vi "BuildM3Sequence.vi"(8 "error in (no error)":errorcluster, 9 "Mode3 Test Properties":T2, 10 "Horizontal T deg":dbl=0.076 format="%#_13g", 11 "Sequence in":refnum<class "Sequence.lvclass">) -> (0 "error out":errorcluster, 2 "PAARD Test Sequence":T4[](array[typedef])=[{"StepType"=enum."Motion", "RF In/Out"=enum."Rx - RF Out", "Module/Raster"=0, "Polarization"=enum."Horizontal", "AO-64 Array"=[], "Position"=[]}, {"StepType"=enum."RasterTest", "RF In/Out"=enum."Tx - RF In", "Module/Raster"=0, "Polarization"=enum."Vertical", "AO-64 Array"=[], "Position"=[]}, {"StepType"=enum."Motion", "RF In/Out"=enum."Rx - RF Out", "Module/Raster"=1, "Polarization"=enum."Horizontal", "AO-64 Array"=[], "Position"=[]}, {"StepType"=enum."RasterTest", "RF In/Out"=enum."Tx - RF In", "Module/Raster"=0, "Polarization"=enum."Vertical", "AO-64 Array"=[], "Position"=[]}, {"StepType"=enum."Motion", "RF In/Out"=enum."Rx - RF Out", "Module/Raster"=2, "Polarization"=enum."Horizontal", "AO-64 Array"=[], "Position"=[]}, {"StepType"=enum."RasterTest", "RF In/Out"=enum."Tx - RF In", "Module/Raster"=0, "Polarization"=enum."Vertical", "AO-64 Array"=[], "Position"=[]}, {"StepType"=enum."Motion", "RF In/Out"=enum."Rx - RF Out", "Module/Raster"=3, "Polarization"=enum."Horizontal", "AO-64 Array"=[], "Position"=[]}, {"StepType"=enum."RasterTest", "RF In/Out"=enum."Tx - RF In", "Module/Raster"=0, "Polarization"=enum."Vertical", "AO-64 Array"=[], "Position"=[]}, {"StepType"=enum."Motion", "RF In/Out"=enum."Rx - RF Out", "Module/Raster"=4, "Polarization"=enum."Horizontal", "AO-64 Array"=[], "Position"=[]}, {"StepType"=enum."RasterTest", "RF In/Out"=enum."Tx - RF In", "Module/Raster"=0, "Polarization"=enum."Vertical", "AO-64 Array"=[], "Position"=[]}, {"StepType"=enum."Motion", "RF In/Out"=enum."Rx - RF Out", "Module/Raster"=5, "Polarization"=enum."Horizontal", "AO-64 Array"=[], "Position"=[]}, {"StepType"=enum."RasterTest", "RF In/Out"=enum."Tx - RF In", "Module/Raster"=0, "Polarization"=enum."Vertical", "AO-64 Array"=[], "Position"=[]}, {"StepType"=enum."Motion", "RF In/Out"=enum."Rx - RF Out", "Module/Raster"=6, "Polarization"=enum."Horizontal", "AO-64 Array"=[], "Position"=[]}, {"StepType"=enum."RasterTest", "RF In/Out"=enum."Tx - RF In", "Module/Raster"=0, "Polarization"=enum."Vertical", "AO-64 Array"=[], "Position"=[]}, {"StepType"=enum."Motion", "RF In/Out"=enum."Rx - RF Out", "Module/Raster"=7, "Polarization"=enum."Horizontal", "AO-64 Array"=[], "Position"=[]}, {"StepType"=enum."RasterTest", "RF In/Out"=enum."Tx - RF In", "Module/Raster"=0, "Polarization"=enum."Vertical", "AO-64 Array"=[], "Position"=[]}, {"StepType"=enum."Motion", "RF In/Out"=enum."Rx - RF Out", "Module/Raster"=8, "Polarization"=enum."Horizontal", "AO-64 Array"=[], "Position"=[]}, {"StepType"=enum."RasterTest", "RF In/Out"=enum."Tx - RF In", "Module/Raster"=0, "Polarization"=enum."Vertical", "AO-64 Array"=[], "Position"=[]}, {"StepType"=enum."Motion", "RF In/Out"=enum."Rx - RF Out", "Module/Raster"=9, "Polarization"=enum."Horizontal", "AO-64 Array"=[], "Position"=[]}, {"StepType"=enum."RasterTest", "RF In/Out"=enum."Tx - RF In", "Module/Raster"=0, "Polarization"=enum."Vertical", "AO-64 Array"=[], "Position"=[]}, {"StepType"=enum."Motion", "RF In/Out"=enum."Rx - RF Out", "Module/Raster"=10, "Polarization"=enum."Horizontal", "AO-64 Array"=[], "Position"=[]}, {"StepType"=enum."RasterTest", "RF In/Out"=enum."Tx - RF In", "Module/Raster"=0, "Polarization"=enum."Vertical", "AO-64 Array"=[], "Position"=[]}, {"StepType"=enum."Motion", "RF In/Out"=enum."Rx - RF Out", "Module/Raster"=11, "Polarization"=enum."Horizontal", "AO-64 Array"=[], "Position"=[]}, {"StepType"=enum."RasterTest", "RF In/Out"=enum."Tx - RF In", "Module/Raster"=0, "Polarization"=enum."Vertical", "AO-64 Array"=[], "Position"=[]}, {"StepType"=enum."Motion", "RF In/Out"=enum."Rx - RF Out", "Module/Raster"=12, "Polarization"=enum."Horizontal", "AO-64 Array"=[], "Position"=[]}, {"StepType"=enum."RasterTest", "RF In/Out"=enum."Tx - RF In", "Module/Raster"=0, "Polarization"=enum."Vertical", "AO-64 Array"=[], "Position"=[]}, {"StepType"=enum."Motion", "RF In/Out"=enum."Rx - RF Out", "Module/Raster"=13, "Polarization"=enum."Horizontal", "AO-64 Array"=[], "Position"=[]}, {"StepType"=enum."RasterTest", "RF In/Out"=enum."Tx - RF In", "Module/Raster"=0, "Polarization"=enum."Vertical", "AO-64 Array"=[], "Position"=[]}, {"StepType"=enum."Motion", "RF In/Out"=enum."Rx - RF Out", "Module/Raster"=14, "Polarization"=enum."Horizontal", "AO-64 Array"=[], "Position"=[]}, {"StepType"=enum."RasterTest", "RF In/Out"=enum."Tx - RF In", "Module/Raster"=0, "Polarization"=enum."Vertical", "AO-64 Array"=[], "Position"=[]}, {"StepType"=enum."Motion", "RF In/Out"=enum."Rx - RF Out", "Module/Raster"=15, "Polarization"=enum."Horizontal", "AO-64 Array"=[], "Position"=[]}, {"StepType"=enum."RasterTest", "RF In/Out"=enum."Tx - RF In", "Module/Raster"=0, "Polarization"=enum."Vertical", "AO-64 Array"=[], "Position"=[]}, {"StepType"=enum."Motion", "RF In/Out"=enum."Rx - RF Out", "Module/Raster"=16, "Polarization"=enum."Horizontal", "AO-64 Array"=[], "Position"=[]}, {"StepType"=enum."RasterTest", "RF In/Out"=enum."Tx - RF In", "Module/Raster"=0, "Polarization"=enum."Vertical", "AO-64 Array"=[], "Position"=[]}, {"StepType"=enum."Motion", "RF In/Out"=enum."Rx - RF Out", "Module/Raster"=17, "Polarization"=enum."Horizontal", "AO-64 Array"=[], "Position"=[]}, {"StepType"=enum."RasterTest", "RF In/Out"=enum."Tx - RF In", "Module/Raster"=0, "Polarization"=enum."Vertical", "AO-64 Array"=[], "Position"=[]}, {"StepType"=enum."Motion", "RF In/Out"=enum."Rx - RF Out", "Module/Raster"=18, "Polarization"=enum."Horizontal", "AO-64 Array"=[], "Position"=[]}, {"StepType"=enum."RasterTest", "RF In/Out"=enum."Tx - RF In", "Module/Raster"=0, "Polarization"=enum."Vertical", "AO-64 Array"=[], "Position"=[]}, {"StepType"=enum."Motion", "RF In/Out"=enum."Rx - RF Out", "Module/Raster"=19, "Polarization"=enum."Horizontal", "AO-64 Array"=[], "Position"=[]}, {"StepType"=enum."RasterTest", "RF In/Out"=enum."Tx - RF In", "Module/Raster"=0, "Polarization"=enum."Vertical", "AO-64 Array"=[], "Position"=[]}, {"StepType"=enum."Finish", "RF In/Out"=enum."Tx - RF In", "Module/Raster"=0, "Polarization"=enum."Vertical", "AO-64 Array"=[], "Position"=[]}], 3 "Sequence out":refnum<class "Sequence.lvclass">, 5 "Axes to Move":T1[](array[typedef]))   [LabVIEW 2018, in "Sequence.lvclass"]
uses:
  Sequence.lvclass
  SequenceSubvis/mWaveTestStep.ctl
  SequenceSubvis/TestStepTypes.ctl
  SequenceSubvis/RF Direction.ctl
  SequenceSubvis/PolarizationSelect.ctl
  APARMainSubvis/VXM Public API/singleAxisMoveDef.ctl
  APARMainSubvis/VXM Public API/mmWaveAxis.ctl
  APARMainSubvis/UI temporary dialogs and VIs/Mode3TestProperties.ctl
  Sequence.lvclass/Sequence.ctl
  <vilib>/Utility/file.llb/Read Delimited Spreadsheet (DBL).vi
panel:
  out "# steps":i32=41
  out "length, bytes":i32=1890 format="%.3p"
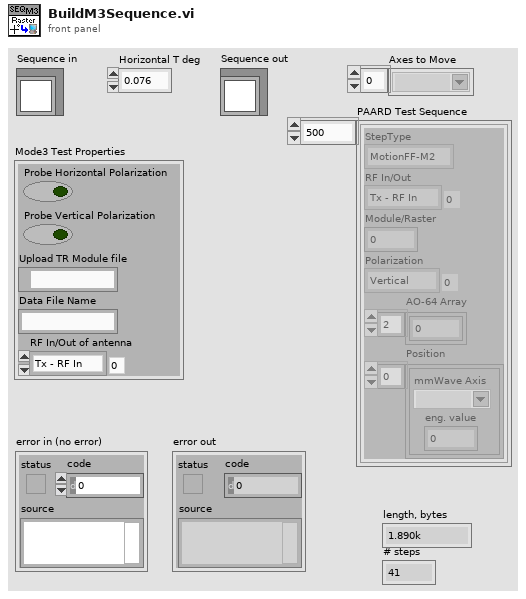
[diagram p1: front panel]
types:
  T1 = typedef "mmWaveAxis.ctl" = string
  T2 = typedef "Mode3TestProperties.ctl" = cluster{"Probe Horizontal Polarization":bool, "Probe Vertical Polarization":bool, "Upload TR Module file":path, "Data File Name":string, "RF In/Out of antenna":T3}
  T3 = typedef "RF Direction.ctl" = enum16{"Tx - RF In", "Rx - RF Out"}
  T4 = typedef "mWaveTestStep.ctl" = cluster{"StepType":T5, "RF In/Out":T3, "Module/Raster":i32, "Polarization":T6, "AO-64 Array":dbl[], "Position":T7[]}
  T5 = typedef "TestStepTypes.ctl" = enum16{"MotionFF-M2", "Motion", "SweepTest", "RasterTest", "Finish", "64ModuleCfg"}
  T6 = typedef "PolarizationSelect.ctl" = enum16{"Vertical", "Horizontal"}
  T7 = typedef "singleAxisMoveDef.ctl" = cluster{"mmWave Axis":T1, "eng. value":dbl}
  T8 = typedef "Mode3FileRowData.ctl" = cluster{"X mm":dbl, "Y mm":dbl, "RT3, degrees":dbl, "sub-file path":path}
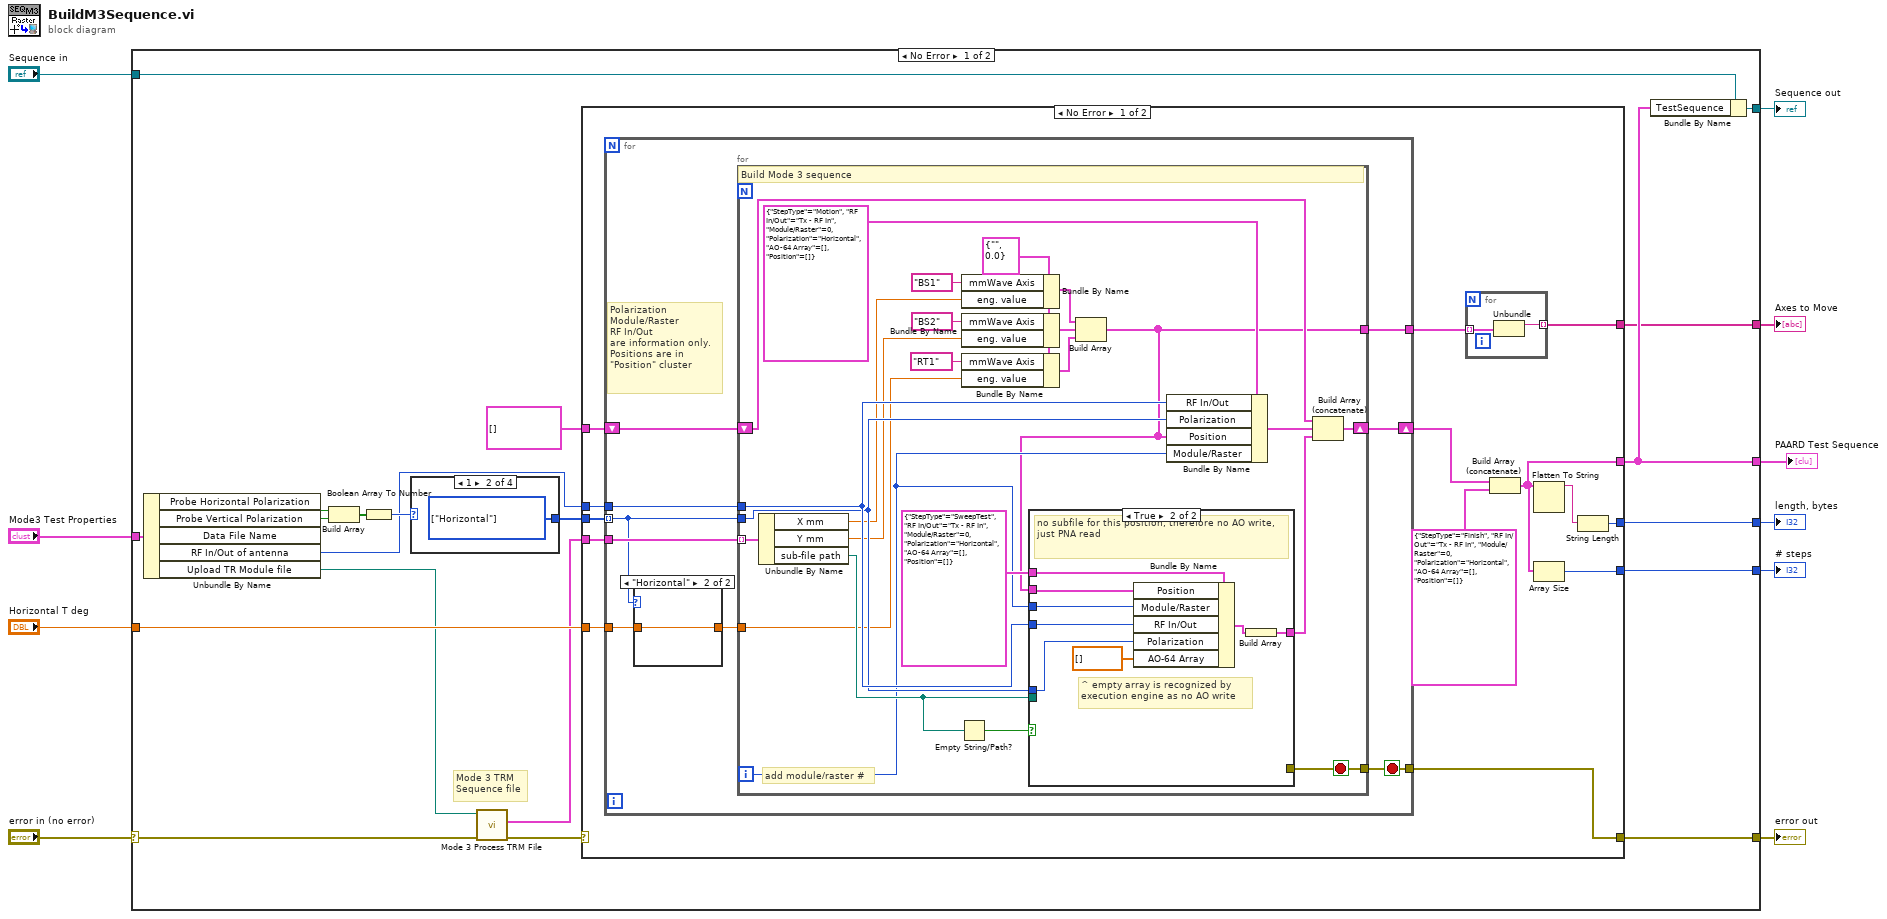
[diagram p0: block diagram]
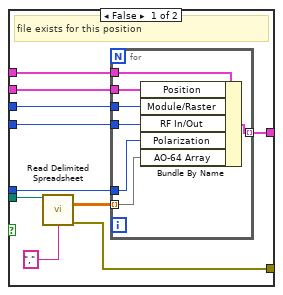
[diagram p2: hidden frame]
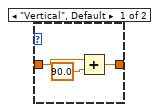
[diagram p3: hidden frame]
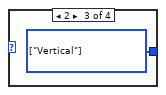
[diagram p6: hidden frame]
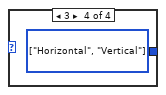
[diagram p7: hidden frame]
diagram:
  n1 = case shown="No Error" "error in (no error)" {
    selector: "error in (no error)" -> [w18 w114]
    tunnel: "Mode3 Test Properties" -> [w29 _]
    tunnel: "Horizontal T deg" -> [w22 _]
    tunnel: [w16 w114] -> w8
    tunnel: "Sequence in" -> [w21 w113]
    tunnel: [w20 w113] -> w6
    tunnel: [w15 _] -> w4
    tunnel: [w14 _] -> w3
    tunnel: [w12 _] -> w2
    tunnel: [w11 _] -> w1
    frame No Error {
      # "Mode 3 TRM\nSequence file"
      n2 = Unbundle By Name(w29) -> ("Probe Horizontal Polarization"=w28:bool, "Probe Vertical Polarization"=w27:bool, "RF In/Out of antenna"=w23:T3, "Upload TR Module file"=w19:path)  [unwired: 1 out]
      n3 = Build Array(w28, w27) -> (w26:bool[])
      n4 = Boolean Array To Number(Boolean array=w26) -> (number=w25:u32)
      n5 = case shown="1" w25 {
        tunnel: [_ w110 w111 w112] -> w24
        frame 0, Default {
          # "should create an \nerror"
        }
        frame 1 {
          w110 = T6[] [enum."Horizontal"] items=["Vertical", "Horizontal"] ("Polarization(s)")
        }
        frame 2 {
          w111 = T6[] [enum."Vertical"] items=["Vertical", "Horizontal"] ("Polarization(s)")
        }
        frame 3 {
          w112 = T6[] [enum."Horizontal", enum."Vertical"] items=["Vertical", "Horizontal"] ("Polarization(s)")
        }
      }
      n6 = call "Mode 3 Process TRM File.vi"("error in (no error)"=w18, "Upload TR Module file"=w19) -> ("error out"=w17:errorcluster, "Mode 3 Steps"=w13:T8[])  [unwired: 7 in, 1 out]
      n7 = case shown="No Error" w17 {
        selector: w17 -> [_ w109]
        tunnel: T4[] [] -> [w44 _]
        tunnel: w24 -> [w43 _]
        tunnel: w23 -> [w42 _]
        tunnel: w22 -> [w41 _]
        tunnel: [w33 w109] -> w16
        tunnel: [w38 _] -> w15
        tunnel: [w37 _] -> w14
        tunnel: [w36 _] -> w12
        tunnel: w13 -> [w34 _]
        tunnel: [w31 _] -> w11
        frame No Error {
          n8 = for {
            tunnel: w42 -> [w50]
            tunnel: w41 -> [w55]
            shift-right: [w53] -> w35
            shift-left: w44 -> [w52]
            tunnel: w43 -> [w49] mode=indexing
            tunnel: w34 -> [w51]
            tunnel: [w48] -> w33
            tunnel: [w47] -> w32
            stop <- w48 stop-if-true
            # "Polarization\nModule/Raster\nRF In/Out\nare information only.\nPositions are in \n\"Position\" cluster"
            n9 = case shown="\"Horizontal\"" w49 {
              tunnel: [w107 w108] -> w54
              tunnel: w55 -> [w106 w108]
              frame "Vertical", Default {
                n10 = Add(x=w106, y=90.0) -> (x+y=w107:dbl)
              }
              frame "Horizontal" {
              }
            }
            n11 = for {
              tunnel: w51 -> [w79] mode=indexing
              shift-right: [w78] -> w53
              shift-left: w52 -> [w68]
              tunnel: w54 -> [w58]
              tunnel: w50 -> [w71]
              tunnel: w49 -> [w70]
              tunnel: [w69] -> w48
              tunnel: [w56] -> w47
              i -> [w57]
              stop <- w69 stop-if-true
              w67 = T7 {"mmWave Axis"="", "eng. value"=0.0} ("Move")
              # "add module/raster #"
              # "Build Mode 3 sequence"
              n12 = Unbundle By Name(w79) -> ("X mm"=w60:dbl, "Y mm"=w59:dbl, "sub-file path"=w72:path)
              n13 = Empty String/Path?(string/path=w72) -> (empty?=w76:bool)
              n14 = Bundle By Name(cluster=w67, "mmWave Axis"=T1 "BS1", "eng. value"=w60) -> (w63:T7)
              n15 = Bundle By Name(cluster=w67, "mmWave Axis"=T1 "BS2", "eng. value"=w59) -> (w62:T7)
              n16 = Bundle By Name(cluster=w67, "mmWave Axis"=T1 "RT1", "eng. value"=w58) -> (w61:T7)
              n17 = Build Array(w63, w62, w61) -> (w56:T7[])
              n18 = case shown="True" w76 {
                tunnel: T4 {"StepType"=enum."SweepTest", "RF In/Out"=enum."Tx - RF In", "Module/Raster"=0, "Polarization"=enum."Horizontal", "AO-64 Array"=[], "Position"=[]} ("Test") -> [w89 w104]
                tunnel: w71 -> [w88 w103]
                tunnel: w70 -> [w86 w102]
                tunnel: [w85 w99] -> w77
                tunnel: w72 -> [w84 _]
                tunnel: w57 -> [w82 w98]
                tunnel: [w81 _] -> w69
                tunnel: w56 -> [w80 w97]
                frame False {
                  # "file exists for this position"
                  n19 = call-poly <vilib>:"Read Delimited Spreadsheet.vi"("file path (dialog if empty)"=w84, "delimiter (\\t)"="," ("delimiter (\\t)")) -> ("all rows"=w87:dbl[][], "error out"=w81:errorcluster)  [unwired: 8 in, 4 out]
                  n20 = for {
                    tunnel: w89 -> [w96]
                    tunnel: w88 -> [w95]
                    tunnel: w87 -> [w94] mode=indexing
                    tunnel: w86 -> [w93]
                    tunnel: [w92] -> w85 mode=indexing
                    tunnel: w82 -> [w91]
                    tunnel: w80 -> [w90]
                    n21 = Bundle By Name(cluster=w96, "Position"=w90, "Module/Raster"=w91, "RF In/Out"=w95, "Polarization"=w93, "AO-64 Array"=w94) -> (w92:T4)
                  }
                }
                frame True {
                  # "^ empty array is recognized by \nexecution engine as no AO write"
                  # "no subfile for this position, therefore no AO write, just PNA read"
                  n22 = Bundle By Name(cluster=w104, "Position"=w97, "Module/Raster"=w98, "RF In/Out"=w103, "Polarization"=w102, "AO-64 Array"=dbl[] []) -> (w100:T4)
                  n23 = Build Array(w100) -> (w99:T4[])
                }
              }
              n24 = Bundle By Name(cluster=T4 {"StepType"=enum."Motion", "RF In/Out"=enum."Tx - RF In", "Module/Raster"=0, "Polarization"=enum."Horizontal", "AO-64 Array"=[], "Position"=[]} ("Test"), "RF In/Out"=w71, "Polarization"=w70, "Position"=w56, "Module/Raster"=w57) -> (w75:T4)
              n25 = Build Array (concatenate)(w68, w75, w77) -> (w78:T4[])
            }
          }
          n26 = for {
            tunnel: w32 -> [w46] mode=indexing
            tunnel: [w45] -> w31 mode=indexing
            n27 = Unbundle(w46) -> ("mmWave Axis"=w45:T1)  [unwired: 1 out]
          }
          n28 = Build Array (concatenate)(w35, T4 {"StepType"=enum."Finish", "RF In/Out"=enum."Tx - RF In", "Module/Raster"=0, "Polarization"=enum."Horizontal", "AO-64 Array"=[], "Position"=[]} ("Test")) -> (w36:T4[])
          n29 = Flatten To String(anything=w36) -> (data string=w40:string)  [unwired: 3 in, 2 out]
          n30 = Array Size(array=w36) -> (size(s)=w38:i32)
          n31 = String Length(string=w40) -> (length=w37:i32)
        }
        frame Error {
        }
      }
      n32 = Bundle By Name(cluster=w21, "TestSequence"=w12) -> (w20:refnum<class "Sequence.lvclass">)
    }
    frame Error {
    }
  }
  "error out" <- w8
  "Sequence out" <- w6
  "PAARD Test Sequence" <- w2
  "length, bytes" <- w3
  "# steps" <- w4
  "Axes to Move" <- w1
